vi "_script_update_doc_txt_stub.vi"() -> ()   [LabVIEW 2014]
uses:
  JKI State Machine++.lvlib
panel:
  out "States":string
  out "appended array":path[](array[path])
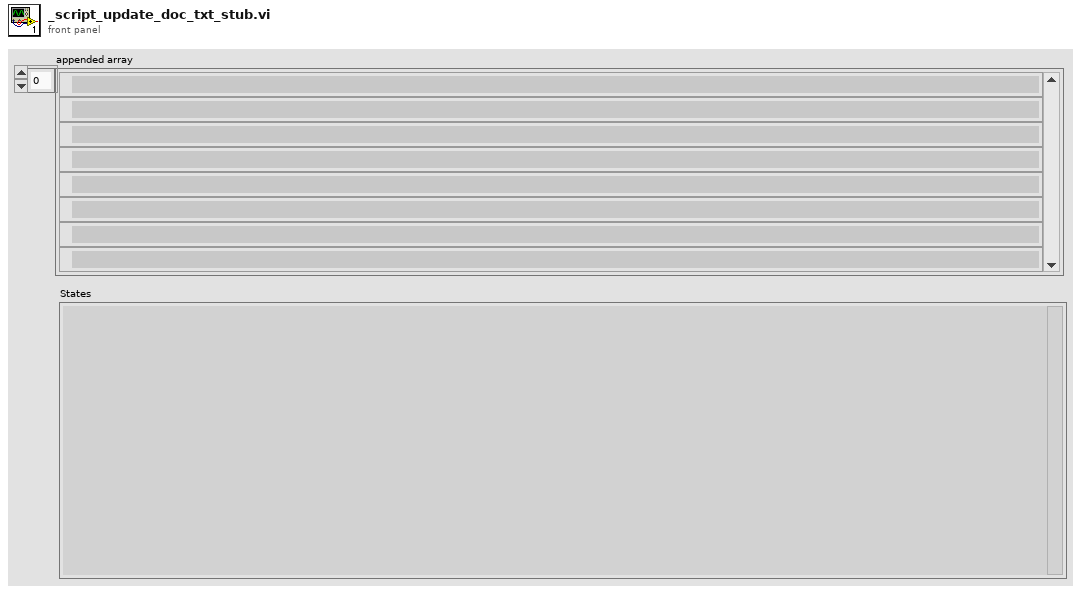
[diagram p1: front panel]
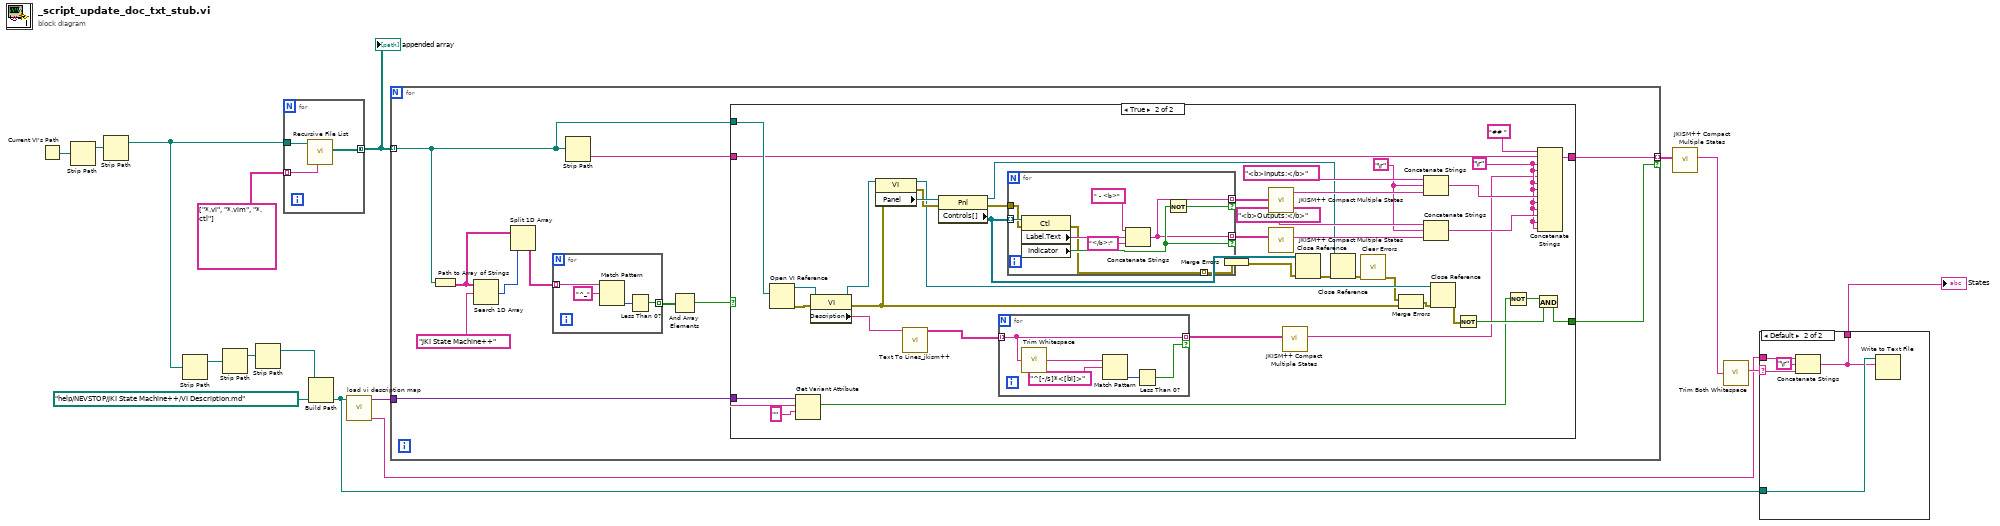
[diagram p0: block diagram]
diagram:
  n1 = Current VI's Path() -> (path=w16:path)
  n2 = Strip Path(path=w16) -> (stripped path=w15:path)  [unwired: 1 out]
  n3 = Strip Path(path=w15) -> (stripped path=w6:path)  [unwired: 1 out]
  n4 = Strip Path(path=w6) -> (stripped path=w11:path)  [unwired: 1 out]
  n5 = Strip Path(path=w11) -> (stripped path=w12:path)  [unwired: 1 out]
  n6 = Strip Path(path=w12) -> (stripped path=w9:path)  [unwired: 1 out]
  n7 = for {
    tunnel: w6 -> [w19]
    tunnel: string[] ["*.vi", "*.vim", "*.ctl"] -> [w18] mode=indexing
    tunnel: [w17] -> w13 mode=concatenating
    n8 = call <vilib>:"Recursive File List.vi"("pattern"=w18, "Folder Path"=w19) -> ("All Files in Dir"=w17:path[])  [unwired: 5 in, 4 out]
  }
  "appended array" <- w13
  n9 = Build Path(base path=w9, name or relative path=path "help/NEVSTOP/JKI State Machine++/VI Description.md" ("Path")) -> (appended path=w4:path)
  n10 = call "load vi description map.vi"("Path"=w4) -> ("text"=w2:string, "variant"=w7:variant)  [unwired: 9 in]
  n11 = for {
    tunnel: w13 -> [w28] mode=indexing
    tunnel: [w30] -> w8 mode=indexing if=w21
    tunnel: w7 -> [w20]
    n12 = Path to Array of Strings(0:w28) -> (2:w25:string[])  [unwired: 1 out]
    n13 = Search 1D Array(1D array=w25, element="JKI State Machine++") -> (index of element=w26:i32)  [unwired: 1 in]
    n14 = Split 1D Array(array=w25, index=w26) -> (second subarray=w24:string[])  [unwired: 1 out]
    n15 = for {
      tunnel: [w32] -> w29 mode=indexing
      tunnel: w24 -> [w31] mode=indexing
      n16 = Match Pattern(string=w31, regular expression="^_") -> (offset past match=w33:i32)  [unwired: 1 in, 3 out]
      n17 = Less Than 0?(x=w33) -> (x < 0?=w32:bool)
    }
    n18 = Strip Path(path=w28) -> (name=w22:string)  [unwired: 1 out]
    n19 = And Array Elements(Boolean array=w29) -> (logical AND=w23:bool)
    n20 = case shown="True" w23 {
      tunnel: [_ w74] -> w30
      tunnel: w28 -> [_ w73]
      tunnel: [_ w64] -> w21
      tunnel: w22 -> [_ w67]
      tunnel: w20 -> [_ w68]
      frame False {
      }
      frame True {
        w43 = "\r"
        w42 = "\r"
        n21 = Open VI Reference(vi path=w73) -> (vi reference=w71:refnum<vi>, error out=w72:errorcluster)  [unwired: 5 in]
        n22 = Get Variant Attribute(Variant=w68, name=w67, default value (empty Variant)="" ("string")) -> (found=w61:bool)  [unwired: 1 in, 3 out]
        n23 = property class="VI"(reference=w71, error in=w72) -> (reference out=w63:refnum<vi>, error out=w38:errorcluster, "Description"=w65:string)
        n24 = property class="VI"(reference=w63, error in=w38) -> (reference out=w44:refnum<vi>, error out=w51:errorcluster, "Panel"=w62:refnum<vi>)
        n25 = call "Text To Lines_jkism++.vi"("string"=w65) -> ("Lines"=w41:string[])  [unwired: 9 in, 1 out]
        n26 = property class="Pnl"(reference=w62, error in=w51) -> (reference out=w45:refnum<vi>, error out=w48:errorcluster, "Controls[]"=w50:refnum<vi>[])
        n27 = for {
          tunnel: w41 -> [w80] mode=indexing
          tunnel: [w80] -> w40 mode=indexing if=w76
          n28 = call <vilib>:"Trim Whitespace.vi"("string"=w80) -> ("trimmed string"=w79:string)  [unwired: 1 in]
          n29 = Match Pattern(string=w79, regular expression="^[-/s]*<[bi]>") -> (offset past match=w77:i32)  [unwired: 1 in, 3 out]
          n30 = Less Than 0?(x=w77) -> (x < 0?=w76:bool)
        }
        n31 = for {
          tunnel: w50 -> [w89] mode=indexing
          tunnel: [w85] -> w59 mode=indexing if=w86
          tunnel: [w85] -> w58 mode=indexing if=w87
          tunnel: w48 -> [w83]
          tunnel: [w82] -> w47 mode=indexing
          n32 = property class="Ctl"(reference=w89, error in=w83) -> (error out=w82:errorcluster, "Label.Text"=w88:string, "Indicator"=w87:bool)  [unwired: 1 out]
          n33 = Concatenate Strings(" - <b>" ("string"), w88, "</b>:" ("string")) -> (w85:string)
          n34 = Not(x=w87) -> (.not. x?=w86:bool)
        }
        n35 = Merge Errors(w47) -> (w46:errorcluster)
        n36 = call "JKISM++ Compact Multiple States.vi"("States in Lines"=w59) -> ("States"=w56:string)  [unwired: 9 in]
        n37 = call "JKISM++ Compact Multiple States.vi"("States in Lines"=w58) -> ("States"=w57:string)  [unwired: 9 in]
        n38 = call "JKISM++ Compact Multiple States.vi"("States in Lines"=w40) -> ("States"=w39:string)  [unwired: 9 in]
        n39 = Close Reference(reference=w50, error in (no error)=w46) -> (error out=w49:errorcluster)
        n40 = Close Reference(reference=w45, error in (no error)=w49) -> (error out=w37:errorcluster)
        n41 = call <vilib>:"Clear Errors.vi"("error in (no error)"=w37) -> ("error out"=w35:errorcluster)  [unwired: 5 in, 1 out]
        n42 = Merge Errors(w35, w38) -> (w36:errorcluster)
        n43 = Concatenate Strings("<b>Inputs:</b>" ("string"), w43, w56) -> (w53:string)
        n44 = Concatenate Strings("<b>Outputs:</b>" ("string"), w43, w57) -> (w52:string)
        n45 = Close Reference(reference=w44, error in (no error)=w36) -> (error out=w70:errorcluster)
        n46 = Not(x=w70) -> (.not. x?=w69:bool)
        n47 = Not(x=w61) -> (.not. x?=w60:bool)
        n48 = And(x=w60, y=w69) -> (x .and. y?=w64:bool)
        n49 = Concatenate Strings("## " ("string"), w67, w42, w42, w39, w42, w42, w53, w42, w42, w52, w42, w42) -> (w74:string)
      }
    }
  }
  n50 = call "JKISM++ Compact Multiple States.vi"("States in Lines"=w8) -> ("States"=w5:string)  [unwired: 9 in]
  n51 = call "Trim Both Whitespace.vi"("string"=w5) -> ("trimmed string"=w3:string)  [unwired: 1 in]
  n52 = case shown="Default" w3 {
    selector: w3 -> [_ w93]
    tunnel: w4 -> [_ w94]
    tunnel: w2 -> [w90 w92]
    tunnel: [w90 w91] -> w1
    frame "" {
    }
    frame Default {
      n53 = Concatenate Strings(w92, "\r", w93) -> (w91:string)
      n54 = Write to Text File(file (use dialog)=w94, text=w91) -> ()  [unwired: 2 in, 3 out]
    }
  }
  "States" <- w1
